vi "RedirectionAnalysis.vi"(8 "error constant":errorcluster) -> (0 "error out":errorcluster)   [LabVIEW 2013]
doc: "Use this template to build a simple state machine design pattern. Each state executes code and determines which state to transition to."
uses:
  Analysis Support/Controls/State.ctl
panel:
  out "Pressure":dbl
  out "selected path":path
  out "Message":string
  in  "Begin":bool
  in  "Exit":bool
  in  "Blank Button":bool
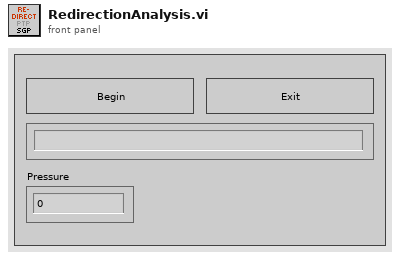
[diagram p1: front panel]
types:
  T1 = typedef "State.ctl" = enum16{"Initialize", "Wait for Event", "Analyze", "Save", "Exit"}
  T2 = enum8{"Enabled", "Disabled", "Disabled and Grayed Out"}
  T3 = enum16{"Left Button", "Center Button", "Right Button", "Window Close"}
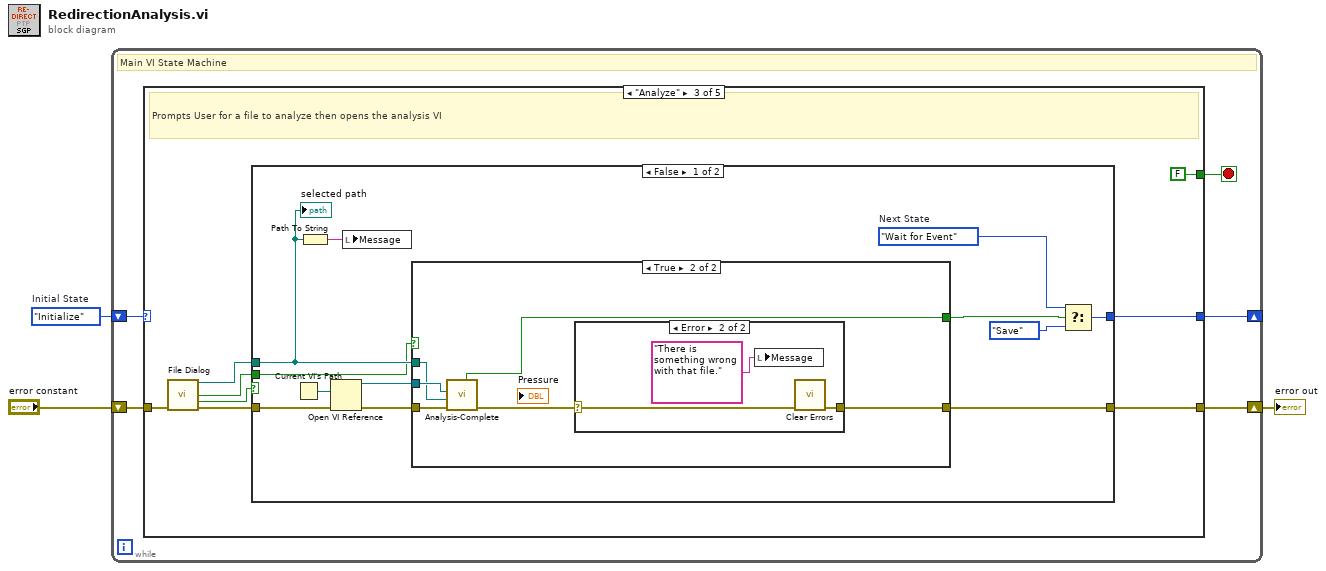
[diagram p0: block diagram]
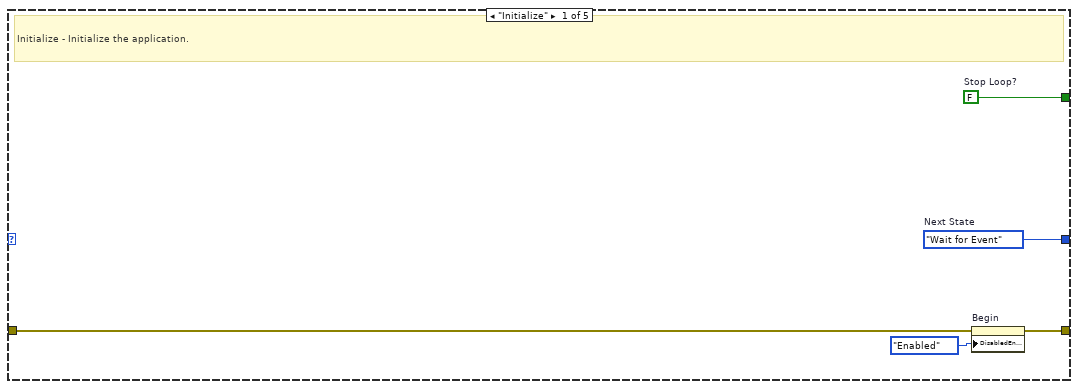
[diagram p2: hidden frame]
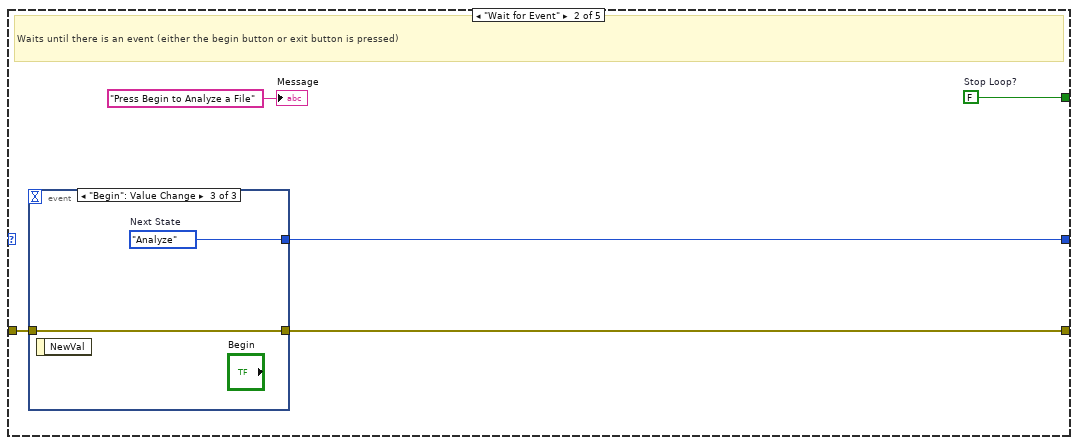
[diagram p3: hidden frame]
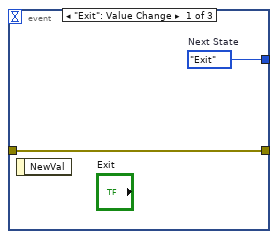
[diagram p4: hidden frame]
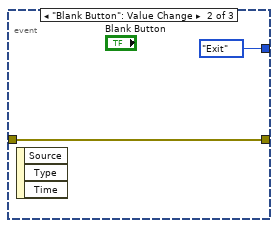
[diagram p5: hidden frame]
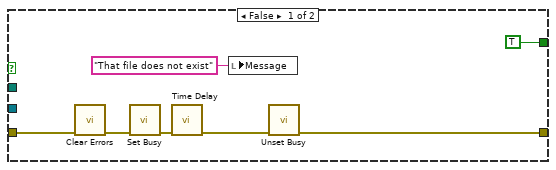
[diagram p6: hidden frame]
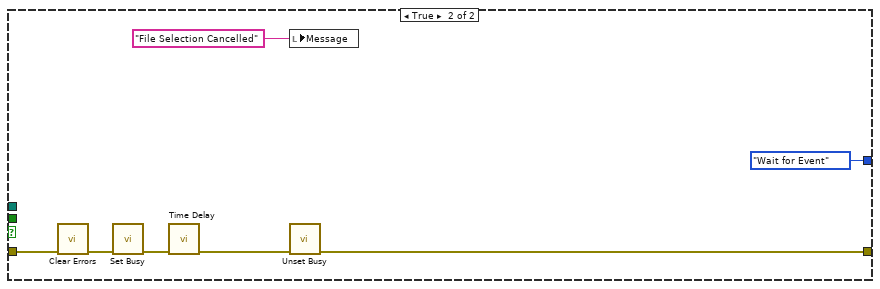
[diagram p8: hidden frame]
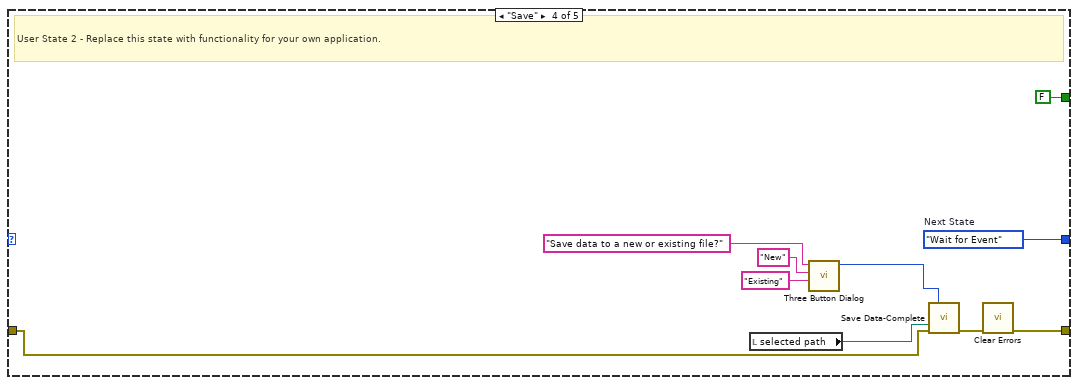
[diagram p9: hidden frame]
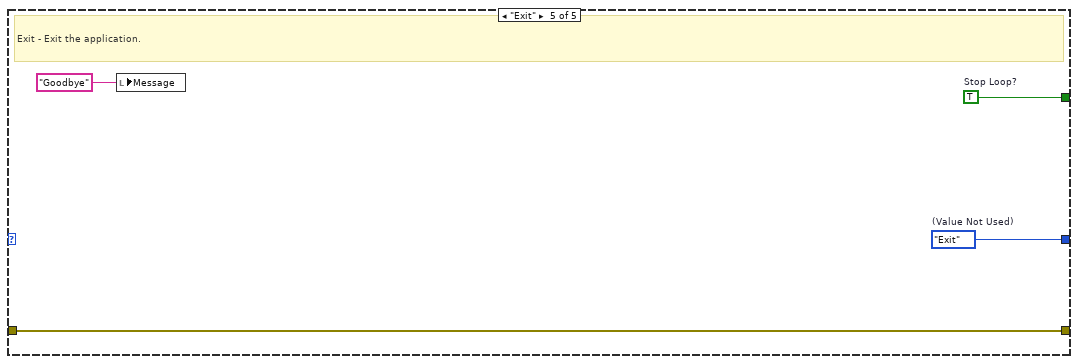
[diagram p10: hidden frame]
diagram:
  w3 = State."Initialize"  # Initial State
  n1 = while {
    shift-right: [w7] -> _
    shift-left: w3 -> [w8]
    shift-right: [w5] -> w1
    shift-left: "error constant" -> [w6]
    stop <- w4 stop-if-true
    # "Main VI State Machine"
    n2 = case shown="\"Analyze\"" w8 {
      tunnel: [w13 w18 w32 w78 w82] -> w7
      tunnel: [w12 w17 FALSE ("Stop Loop?") FALSE ("Stop Loop?") w81] -> w4
      tunnel: w6 -> [w11 w16 w29 w75 w80]
      tunnel: [w9 w15 w30 w70 w80] -> w5
      frame "Initialize" {
        w12 = FALSE  # Stop Loop?
        w13 = State."Wait for Event"  # Next State
        # "Initialize - Initialize the application."
        n3 = property on="Begin" class="Bool"(error in=w11, "DisabledEnum"=T2."Enabled" ("Disabled")) -> (error out=w9:errorcluster)  [unwired: 1 in, 1 out]
      }
      frame "Wait for Event" {
        w17 = FALSE  # Stop Loop?
        # "Waits until there is an event (either the begin button or exit button is pressed)"
        n4 = event shown="[2] \"Begin\": Value Change" {
          selector: _ -> [_ _ _]
          dyn-events: _ -> [_ _ _]
          timeout: _ -> [_ _ _]
          tunnel: [w20 State."Exit" ("Next State") w24] -> w18
          tunnel: w16 -> [w19 w22 w23]
          tunnel: [w19 w22 w23] -> w15
          event "Exit": Value Change {
            w20 = State."Exit"  # Next State
            n5 = event-data() -> ()  [unwired: 1 in, 1 out]
          }
          event "Blank Button": Value Change {
            n6 = event-data() -> ()  [unwired: 1 in, 3 out]
          }
          event "Begin": Value Change {
            w24 = State."Analyze"  # Next State
            n7 = event-data() -> ()  [unwired: 1 in, 1 out]
          }
        }
        "Message" <- "Press Begin to Analyze a File" ("String")
      }
      frame "Analyze" {
        # "Prompts User for a file to analyze then opens the analysis VI"
        n8 = call "File Dialog"("error in"=w29) -> ("selected path"=w26:path, "exists"=w27:bool, "cancelled"=w25:bool, "error out"=w28:errorcluster)  [unwired: 11 in]
        n9 = case shown="False" w25 {
          tunnel: [w36 State."Wait for Event" ("Next State")] -> w32
          tunnel: [w44 w62] -> w30
          tunnel: w28 -> [w42 w67]
          tunnel: w27 -> [w37 _]
          tunnel: w26 -> [w39 _]
          frame False {
            w35 = State."Wait for Event"  # Next State
            n10 = Current VI's Path() -> (path=w43:path)
            n11 = Path To String(path=w39) -> (string=w38:string)
            n12 = Open VI Reference(vi path=w43, error in (no error)=w42) -> (vi reference=w40:refnum<vi>, error out=w41:errorcluster)  [unwired: 4 in]
            n13 = local write "Message"(w38) -> ()
            n14 = case shown="True" w37 {
              tunnel: [w48 w55] -> w44
              tunnel: w39 -> [_ w52]
              tunnel: w41 -> [w46 w57]
              tunnel: w40 -> [_ w53]
              tunnel: [TRUE ("error?") w54] -> w33
              frame False {
                n15 = call <vilib>:"Clear Errors.vi"("error in (no error)"=w46) -> ("error out"=w47:errorcluster)  [unwired: 6 in]
                n16 = call <vilib>:"Set Busy.vi"("error in (no error)"=w47) -> ("error out"=w50:errorcluster)  [unwired: 9 in, 1 out]
                n17 = call "Time Delay"("error in (no error)"=w50) -> ("error out"=w49:errorcluster)  [unwired: 10 in]
                n18 = local write "Message"("That file does not exist" ("Message")) -> ()
                n19 = call <vilib>:"Unset Busy.vi"("error in (no error)"=w49) -> ("error out"=w48:errorcluster)  [unwired: 10 in]
              }
              frame True {
                n20 = call "Analysis-Complete.vi"("error in (no error)"=w57, "selected path"=w52, "VI reference"=w53) -> ("error out"=w56:errorcluster, "error?"=w54:bool)  [unwired: 4 in, 3 out]
                n21 = case shown="Error" w56 {
                  selector: w56 -> [w58 w60]
                  tunnel: [w58 w59] -> w55
                  frame No Error {
                  }
                  frame Error {
                    n22 = local write "Message"("There is something wrong with that file." ("Message")) -> ()
                    n23 = call <vilib>:"Clear Errors.vi"("error in (no error)"=w60) -> ("error out"=w59:errorcluster)  [unwired: 6 in]
                  }
                }
              }
            }
            n24 = Select(t=w35, s=w33, f=State."Save") -> (s? t:f=w36:T1)
            "selected path" <- w39
          }
          frame True {
            n25 = call <vilib>:"Clear Errors.vi"("error in (no error)"=w67) -> ("error out"=w64:errorcluster)  [unwired: 6 in]
            n26 = call <vilib>:"Set Busy.vi"("error in (no error)"=w64) -> ("error out"=w65:errorcluster)  [unwired: 9 in, 1 out]
            n27 = call "Time Delay"("error in (no error)"=w65) -> ("error out"=w63:errorcluster)  [unwired: 10 in]
            n28 = local write "Message"("File Selection Cancelled" ("Message")) -> ()
            n29 = call <vilib>:"Unset Busy.vi"("error in (no error)"=w63) -> ("error out"=w62:errorcluster)  [unwired: 10 in]
          }
        }
      }
      frame "Save" {
        w78 = State."Wait for Event"  # Next State
        # "User State 2 - Replace this state with functionality for your own application."
        n30 = local read "selected path"() -> (w69:path)
        n31 = call <vilib>:"Three Button Dialog.vi"("Center Button Text (\"No\")"="Existing" ("T button name (\"OK\")"), "Left Button Text (\"Yes\")"="New" ("F button name (\"Cancel\")"), "message"="Save data to a new or existing file?") -> ("Which Button?"=w74:T3)  [unwired: 8 in]
        n32 = call "Save Data-Complete.vi"("Which Button?"=w74, "selected path"=w69, "error in (no error)"=w75) -> ("error out"=w71:errorcluster)  [unwired: 12 in]
        n33 = call <vilib>:"Clear Errors.vi"("error in (no error)"=w71) -> ("error out"=w70:errorcluster)  [unwired: 6 in]
      }
      frame "Exit" {
        w81 = TRUE  # Stop Loop?
        w82 = State."Exit"  # (Value Not Used)
        # "Exit - Exit the application."
        n34 = local write "Message"("Goodbye" ("Message")) -> ()
      }
    }
  }
  "error out" <- w1
